vi "Debounce.vi"(11 "booleanIn":bool) -> (3 "booleanOut":bool)   [LabVIEW 2018]
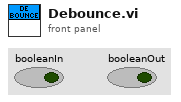
[diagram p1: front panel]
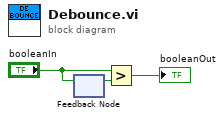
[diagram p0: block diagram]
diagram:
  n1 = feedback #1() -> (w2:bool)  [unwired: 1 in]
  n2 = feedback-in #1("booleanIn") -> ()
  n3 = Greater?(x="booleanIn", y=w2) -> (0:→"booleanOut":bool)
